vi "test_csm_lumikki_instron_moveToSetpoint.vi"   [LabVIEW 2009]
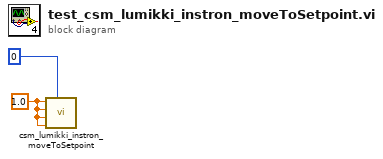
[diagram p0: block diagram]
diagram:
  w1 = 1.0 ("Set Point")
  n1 = call "csm_lumikki_instron_moveToSetpoint.vi"("ChannelInt"=0, "Ramp Rate"=w1, "Ramp Amplitude"=w1, "Set Point Time"=w1, "Set Point"=w1) -> ()  [unwired: 7 in]
